vi "Plant Identification 2.vi"() -> ()   [LabVIEW 2015]
uses:
  <vilib>/measure/NI_MABase.lvlib
panel:
  in  "Amplitude (Vpp)":dbl(slide)=4.5 scale=0.0..9.0
  in  "Frequency (Hz)":dbl(slide)=0.5 scale=0.0..1.0
  in  "Offset (Vdc)":dbl(slide)=4.5 scale=0.0..5.0
  out "Speed (rps)":dynamicdata(graph)
  in  "stop (F)":bool
  # "Square Wave Parameters"
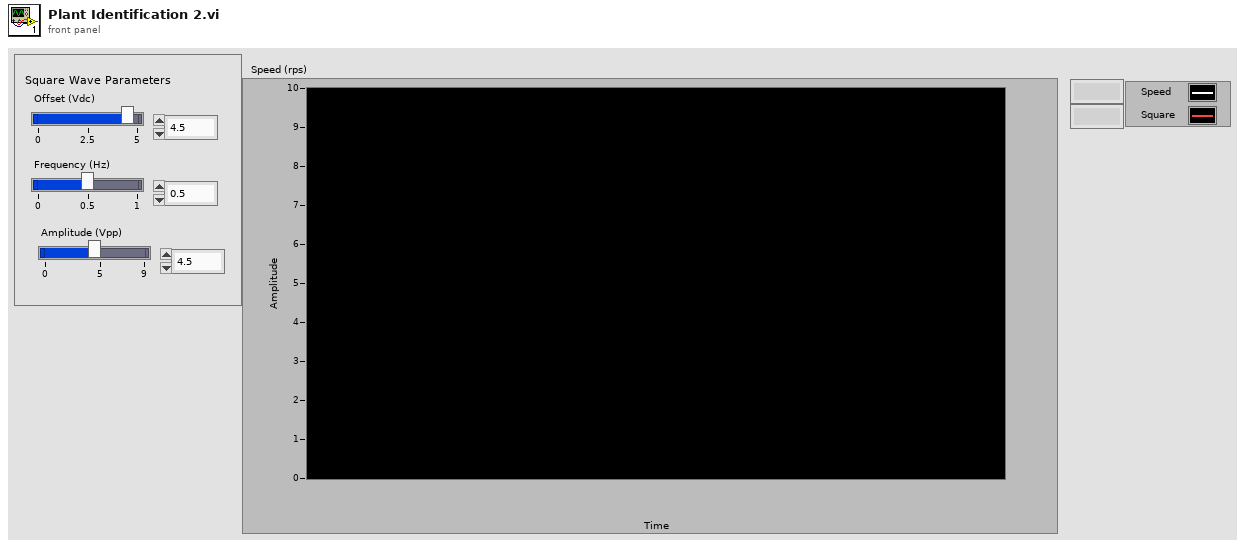
[diagram p1: front panel]
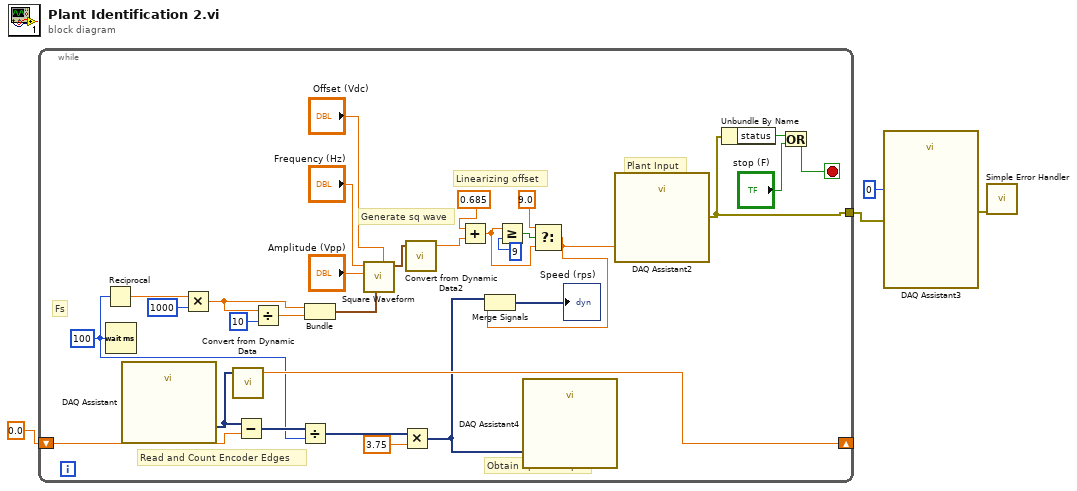
[diagram p0: block diagram]
diagram:
  n1 = while {
    shift-right: [w34] -> _
    shift-left: 0.0 -> [w33]
    tunnel: [w29] -> w3
    stop <- w28 stop-if-true
    w17 = 100
    # "Linearizing offset"
    # "Fs"
    # "Obtain Speed in rps"
    # "Read and Count Encoder Edges"
    # "Plant Input"
    # "Generate sq wave"
    n2 = Reciprocal(x=w17) -> (1/x=w19:dbl)
    n3 = Wait (ms)(milliseconds to wait=w17) -> ()  [unwired: 1 out]
    n4 = call "DAQ Assistant"() -> ("data"=w25:dynamicdata)  [unwired: 16 in, 3 out]
    n5 = Multiply(x=w19, y=1000) -> (x*y=w14:dbl)
    n6 = call "Convert from Dynamic Data"("Dynamic Data Type"=w25) -> ("Scalar"=w34:dbl)  [unwired: 3 in]
    n7 = Subtract(x=w25, y=w33) -> (x-y=w32:dynamicdata)
    n8 = Divide(x=w14, y=10) -> (x/y=w12:dbl)
    n9 = Divide(x=w32, y=w17) -> (x/y=w31:dynamicdata)
    n10 = Bundle(w14, w12) -> (w15:cluster{dbl, dbl})  [unwired: 1 in]
    n11 = call <vilib>:"Square Waveform.vi"("offset"="Offset (Vdc)", "sampling info"=w15, "amplitude"="Amplitude (Vpp)", "frequency"="Frequency (Hz)") -> ("signal out"=w22:waveform(dbl))  [unwired: 6 in, 1 out]
    n12 = Multiply(x=w31, y=3.75) -> (x*y=w23:dynamicdata)
    n13 = call "Convert from Dynamic Data2"("Dynamic Data Type"=w22) -> ("Scalar"=w11:dbl)  [unwired: 3 in]
    n14 = Add(x=0.685, y=w11) -> (x+y=w6:dbl)
    n15 = Greater Or Equal?(x=w6, y=9) -> (x >= y?=w8:bool)
    n16 = call "DAQ Assistant4"("data"=w23) -> ()  [unwired: 17 in, 2 out]
    n17 = Select(t=9.0, s=w8, f=w6) -> (s? t:f=w5:dbl)
    n18 = Merge Signals(w23, w5) -> (→"Speed (rps)":dynamicdata)
    n19 = call "DAQ Assistant2"("data"=w5) -> ("error out"=w29:errorcluster)  [unwired: 17 in, 1 out]
    n20 = Unbundle By Name(w29) -> ("status"=w26:bool)
    n21 = Or(x=w26, y="stop (F)") -> (x .or. y?=w28:bool)
  }
  n22 = call "DAQ Assistant3"("data"=0, "error in"=w3) -> ("error out"=w1:errorcluster)  [unwired: 16 in, 1 out]
  n23 = call <vilib>:"Simple Error Handler.vi"("error in (no error)"=w1) -> ()  [unwired: 4 in, 5 out]
